vi "SelectVideoMode.vi"(8 "error in (no error)":errorcluster, 11 "Refnum in":T1) -> (0 "error out":errorcluster, 3 "Refnum out":T1)   [LabVIEW 2018]
uses:
  <vilib>/userdefined/High Color/IMAQdx.ctl
  <vilib>/vision/driver/NI_Vision_Acquisition_Software.lvlib
  <resource>/objmgr/imaqdx.rc
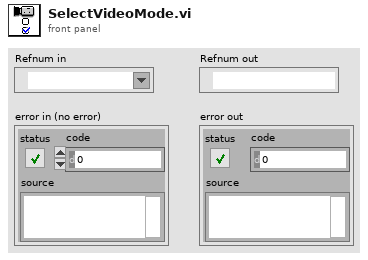
[diagram p1: front panel]
types:
  T1 = typedef "IMAQdx.ctl" = refnum<k21>
  T2 = cluster{"Video Mode":u32, "Video Mode Name":string}[]
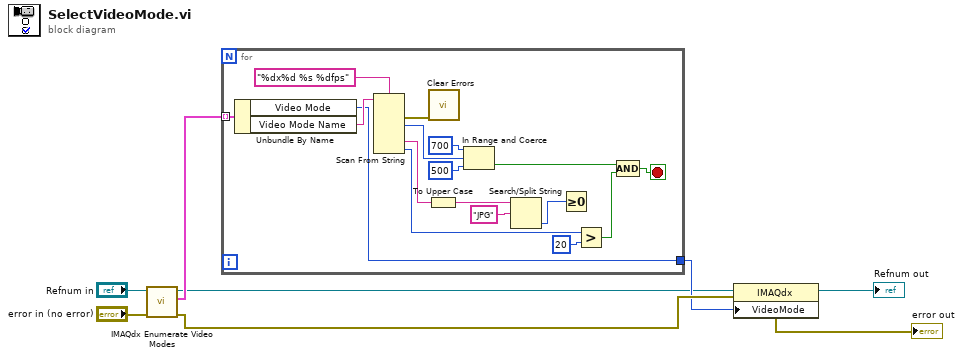
[diagram p0: block diagram]
diagram:
  n1 = call <vilib>:"IMAQdx Enumerate Video Modes.vi"("error in"="error in (no error)", "Session In"="Refnum in") -> ("error out"=w7:errorcluster, "Video Modes"=w5:T2, "Session Out"=w2:T1)  [unwired: 6 in, 1 out]
  n2 = for {
    tunnel: w5 -> [w23] mode=indexing
    tunnel: [w10] -> w6
    stop <- w9 stop-if-true
    n3 = Unbundle By Name(w23) -> ("Video Mode"=w10:u32, "Video Mode Name"=w22:string)
    n4 = Scan From String(format string="%dx%d %s %dfps", input string=w22) -> (error out=w24:errorcluster, output 1=w15:i32, output 3=w21:string, output 4=w17:i32)  [unwired: 7 in, 2 out]
    n5 = To Upper Case(1:w21) -> (0:w19:string)
    n6 = call <vilib>:"Clear Errors.vi"("error in (no error)"=w24) -> ()  [unwired: 5 in, 2 out]
    n7 = In Range and Coerce(upper limit=700, x=w15, lower limit=500) -> (In Range?=w11:bool)  [unwired: 1 out]
    n8 = Search/Split String(string=w19, search string/char (-)="JPG") -> (offset of match=w18:i32)  [unwired: 1 in, 2 out]
    n9 = Greater Or Equal To 0?(x=w18) -> ()  [unwired: 1 out]
    n10 = Greater?(x=w17, y=20) -> (0:w12:bool)
    n11 = Compound Arithmetic op=AND(w11, w12) -> (w9:bool)
  }
  n12 = property class="IMAQdx"(reference=w2, error in=w7, "VideoMode"=w6) -> (reference out=→"Refnum out":T1, error out=→"error out":errorcluster)
